vi "Test Transcriptor LabVIEW to C code 2.vi"() -> ()   [LabVIEW 2014]
panel:
  in  "vi path":path=path "C:/Users/ljagos/Documents/LabVIEW/LabVIEW-Universal-Transcriptor/Test/Examples For Parsing/Example Cluster 1.vi"
  out "resulting string":string
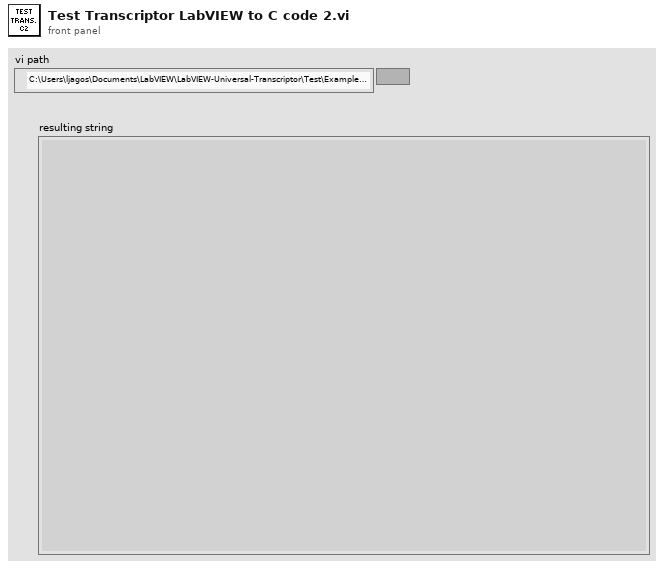
[diagram p1: front panel]
types:
  T1 = cluster{"Defines":string[], "Includes":string[], "C code":string}
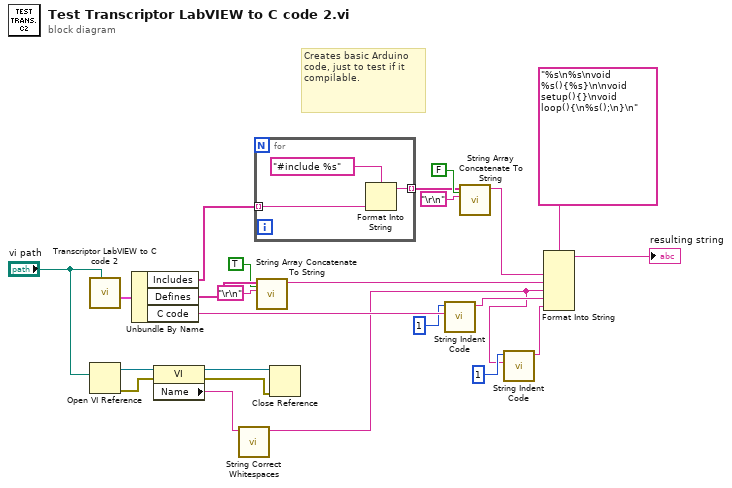
[diagram p0: block diagram]
diagram:
  # "Creates basic Arduino code, just to test if it compilable."
  n1 = call "Transcriptor LabVIEW to C code 2.vi"("vi path"="vi path") -> ("output cluster"=w24:T1)  [unwired: 7 in, 3 out]
  n2 = Open VI Reference(vi path="vi path") -> (vi reference=w11:refnum<vi>, error out=w13:errorcluster)  [unwired: 5 in]
  n3 = Unbundle By Name(w24) -> ("Includes"=w15:string[], "Defines"=w22:string[], "C code"=w6:string)
  n4 = property class="VI"(reference=w11, error in=w13) -> (reference out=w10:refnum<vi>, error out=w8:errorcluster, "Name"=w9:string)
  n5 = call "String Correct Whitespaces.vi"("String in"=w9) -> ("String out"=w2:string)  [unwired: 10 in]
  n6 = for {
    tunnel: w15 -> [w26] mode=indexing
    tunnel: [w25] -> w14 mode=indexing
    n7 = Format Into String(format string="#include %s", w26) -> (resulting string=w25:string)  [unwired: 2 in, 1 out]
  }
  n8 = call "String Array Concatenate To String.vi"("insert last delimiter?"=TRUE, "Delimiter char"="\r\n", "Array String In"=w22) -> ("String"=w20:string)  [unwired: 8 in]
  n9 = Close Reference(reference=w10, error in (no error)=w8) -> ()  [unwired: 1 out]
  n10 = call "String Indent Code.vi"("complete code"=w6, "actual nested level"=1) -> ("indented code"=w5:string)  [unwired: 9 in]
  n11 = call "String Array Concatenate To String.vi"("insert last delimiter?"=FALSE, "Delimiter char"="\r\n", "Array String In"=w14) -> ("String"=w16:string)  [unwired: 8 in]
  n12 = call "String Indent Code.vi"("complete code"=w2, "actual nested level"=1) -> ("indented code"=w1:string)  [unwired: 9 in]
  n13 = Format Into String(format string="%s\n%s\nvoid %s(){%s}\n\nvoid setup(){}\nvoid loop(){\n%s();\n}\n", w16, w20, w2, w5, w1) -> (resulting string=→"resulting string":string)  [unwired: 2 in, 1 out]
